vi "获取本机IP.vi"() -> (0 "IP3":string, 1 "IP地址 2":string, 3 "IP地址":string)   [LabVIEW 2010]
panel:
  out "MAC地址":string
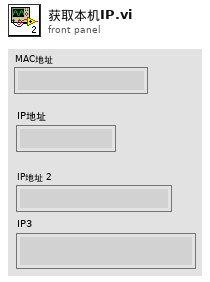
[diagram p1: front panel]
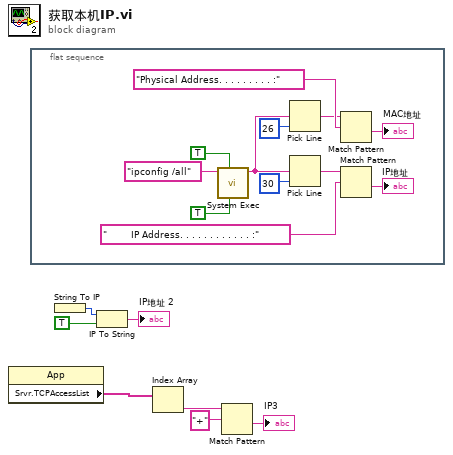
[diagram p0: block diagram]
diagram:
  n1 = property class="App"() -> ("Srvr.TCPAccessList"=w4:string[])  [unwired: 2 in, 2 out]
  n2 = flat-sequence {
    frame #0 {
      n3 = call <vilib>:"System Exec.vi"("run minimized? (F)"=TRUE, "wait until completion? (T)"=TRUE, "command line"="ipconfig /all") -> ("standard output"=w11:string)  [unwired: 3 in, 5 out]
      n4 = Pick Line(multi-line string=w11, line index=26) -> (output string=w13:string)  [unwired: 1 out]
      n5 = Pick Line(multi-line string=w11, line index=30) -> (output string=w9:string)  [unwired: 1 out]
      n6 = Match Pattern(string=w13, regular expression="Physical Address. . . . . . . . . :") -> (after substring=→"MAC地址":string)  [unwired: 4 out]
      n7 = Match Pattern(string=w9, regular expression="        IP Address. . . . . . . . . . . . :") -> (after substring=→"IP地址":string)  [unwired: 4 out]
    }
  }
  n8 = String To IP() -> (0:w5:u32)  [unwired: 1 out]
  n9 = IP To String(1:TRUE ("dot notation? (F)"), 2:w5) -> (0:→"IP地址 2":string)
  n10 = Index Array(array=w4) -> (element=w3:string)  [unwired: 1 in]
  n11 = Match Pattern(string=w3, regular expression="+" ("正则表达式")) -> (after substring=→"IP3":string)  [unwired: 1 in, 3 out]
